vi "pp2_log_toString_sessionList.vi"(11 "Session List in":u8[](array[numeric]) min=1 step=1) -> (3 "spreadsheet string":string)   [LabVIEW 2013]
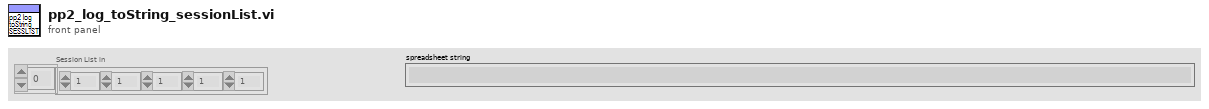
[diagram p1: front panel]
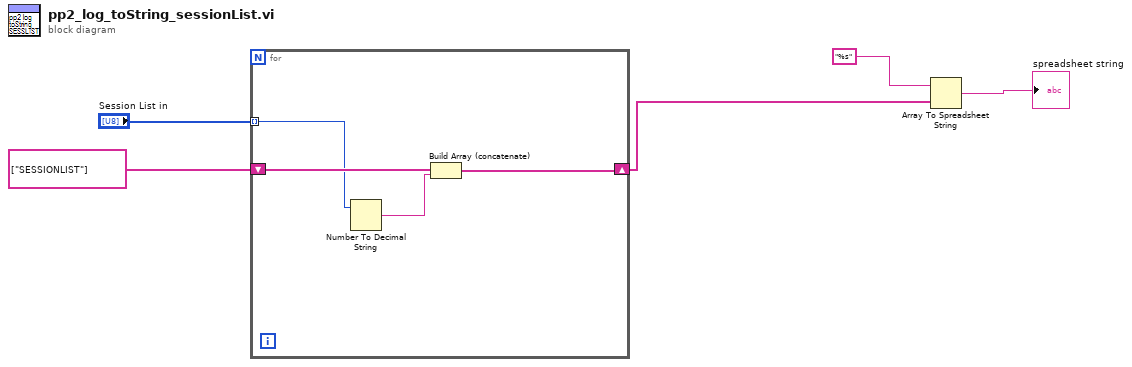
[diagram p0: block diagram]
diagram:
  n1 = for {
    shift-right: [w6] -> w1
    shift-left: string[] ["SESSIONLIST"] -> [w9]
    tunnel: "Session List in" -> [w8] mode=indexing
    n2 = Number To Decimal String(number=w8) -> (decimal integer string=w7:string)  [unwired: 1 in]
    n3 = Build Array (concatenate)(w9, w7) -> (w6:string[])
  }
  n4 = Array To Spreadsheet String(array=w1, 3:"%s" ("format string")) -> (spreadsheet string=→"spreadsheet string":string)  [unwired: 1 in]
